vi "Set_Sweep_Parameter.vi"(5 "MPM":refnum<k24>[](array[refnum]), 6 "布尔":bool, 7 "OSU":refnum<k24>, 8 "错误输入（无错误）":errorcluster, 9 "TSL_OSUport":dbl, 10 "TSLSweepItem":T1, 11 "SPU":refnum<k24>) -> (0 "错误输出":errorcluster, 1 "MPM out":refnum<k24>[](array[refnum]), 2 "OSU out":refnum<k24>, 3 "SPU out":refnum<k24>)   [LabVIEW 2017]
uses:
  D:/test/FULLband-sts/Fullband_Sample/DLL/InstrumentDLL.dll
  DLL/InstrumentDLL.dll
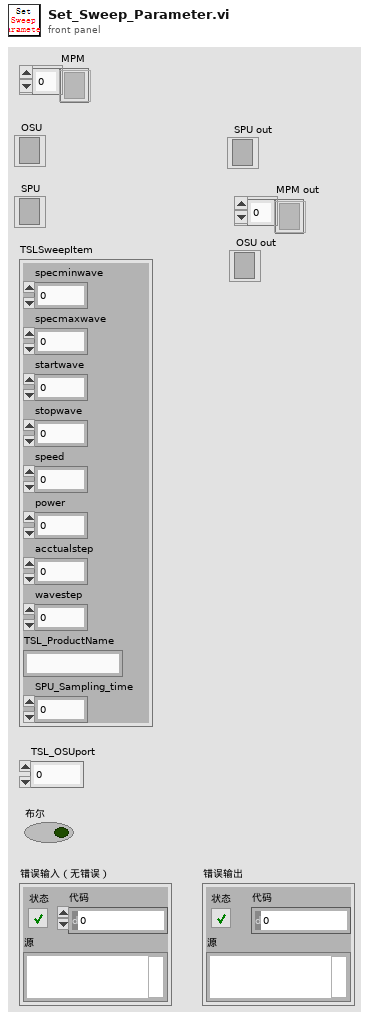
[diagram p1: front panel]
types:
  T1 = cluster{"specminwave":dbl, "specmaxwave":dbl, "startwave":dbl, "stopwave":dbl, "speed":dbl, "power":dbl, "acctualstep":dbl, "wavestep":dbl, "TSL_ProductName":string, "SPU_Sampling_time":dbl}
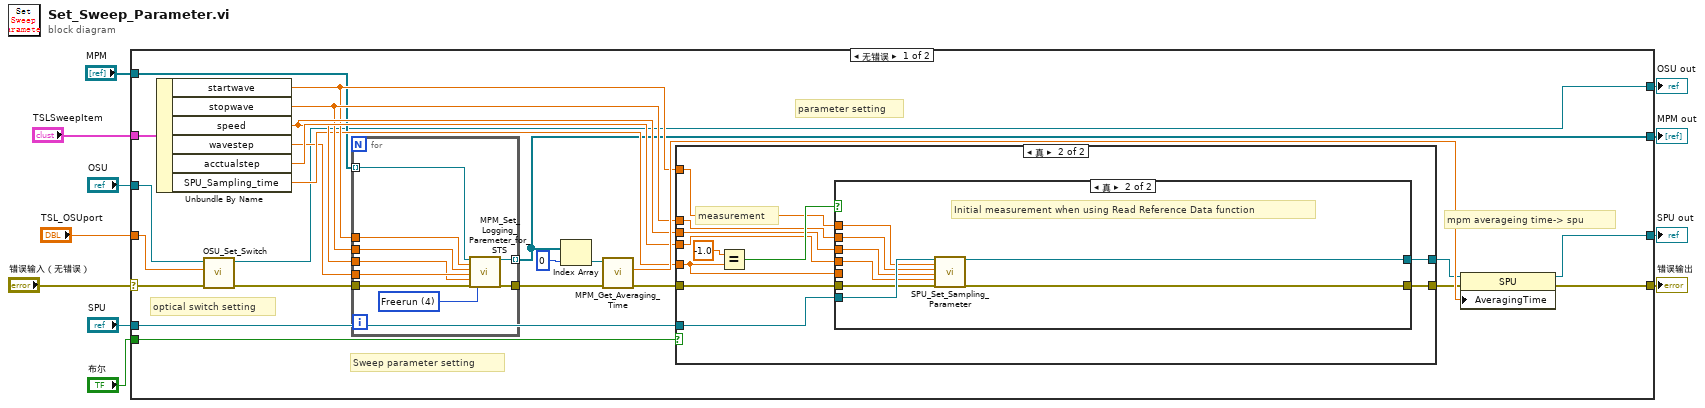
[diagram p0: block diagram]
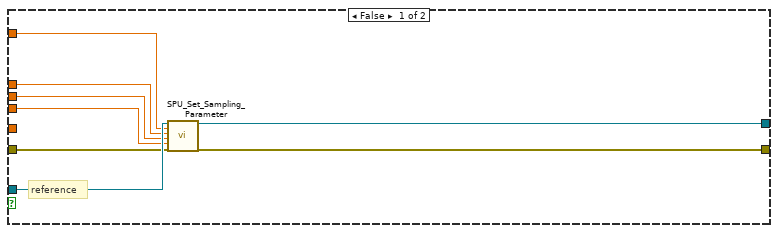
[diagram p2: hidden frame]
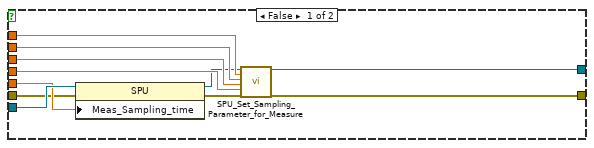
[diagram p3: hidden frame]
diagram:
  n1 = case shown="无错误" "错误输入（无错误）" {
    selector: "错误输入（无错误）" -> [w15 w87]
    tunnel: [w36 w87] -> w11
    tunnel: "SPU" -> [w27 w86]
    tunnel: "布尔" -> [w25 _]
    tunnel: "MPM" -> [w21 w84]
    tunnel: "TSL_OSUport" -> [w18 _]
    tunnel: "OSU" -> [w17 w85]
    tunnel: "TSLSweepItem" -> [w16 _]
    tunnel: [w14 w86] -> w3
    tunnel: [w13 w84] -> w2
    tunnel: [w12 w85] -> w1
    frame No Error {
      # "mpm averageing time-> spu"
      # "parameter setting"
      # "Sweep parameter setting"
      # "optical switch setting"
      n2 = Unbundle By Name(w16) -> ("startwave"=w29:dbl, "stopwave"=w30:dbl, "speed"=w31:dbl, "wavestep"=w20:dbl, "acctualstep"=w32:dbl, "SPU_Sampling_time"=w26:dbl)
      n3 = call "OSU_Set_Switch.vi"("error in (no error)"=w15, "channel"=w18, ".NET Reference in"=w17) -> ("error out"=w19:errorcluster, "Reference out"=w12:refnum<k24>)  [unwired: 7 in]
      n4 = for {
        tunnel: w19 -> [w83]
        tunnel: w21 -> [w82] mode=indexing
        tunnel: w29 -> [w81]
        tunnel: w30 -> [w80]
        tunnel: w20 -> [w79]
        tunnel: w31 -> [w78]
        tunnel: [w76] -> w24
        tunnel: [w75] -> w13 mode=indexing
        w77 = 4 items=["ManualRangeConstant", "ManualRangeSweep", "AutoRangeConstant", "AutoRangeSweep", "Freerun"] ("mode")
        n5 = call "MPM_Set_Logging_Paremeter_for_STS.vi"(".NET Reference in"=w82, "startwave"=w81, "stopwave"=w80, "wavestep"=w79, "speed"=w78, "error in (no error)"=w83, "mode"=w77) -> ("Reference out"=w75:refnum<k24>, "error out"=w76:errorcluster)  [unwired: 11 in]
      }
      n6 = Index Array(array=w13, index=0 ("索引")) -> (element=w23:refnum<k24>)
      n7 = call "MPM_Get_Averaging_Time.vi"("error in (no error)"=w24, ".NET Reference in"=w23) -> ("error out"=w28:errorcluster, "time out"=w35:dbl)  [unwired: 7 in, 1 out]
      n8 = case shown="真" w25 {
        tunnel: w26 -> [_ w46]
        tunnel: w27 -> [w44 w54]
        tunnel: w28 -> [w43 w50]
        tunnel: w29 -> [w42 w53]
        tunnel: w30 -> [w41 w49]
        tunnel: w31 -> [w40 w52]
        tunnel: w32 -> [w39 w51]
        tunnel: [w37 w48] -> w33
        tunnel: [w38 w47] -> w34
        frame False {
          # "reference"
          n9 = call "SPU_Set_Sampling_Parameter.vi"("引用"=w44, "startwave"=w42, "stopwave"=w41, "speed"=w40, "triggerstep"=w39, "错误输入（无错误）"=w43) -> ("引用输出"=w38:refnum<k24>, "error IO"=w37:errorcluster)  [unwired: 12 in]
        }
        frame True {
          # "measurement"
          n10 = Equal?(x=-1.0, y=w46) -> (x = y?=w55:bool)
          n11 = case shown="真" w55 {
            tunnel: w54 -> [w60 w74]
            tunnel: w53 -> [w66 w70]
            tunnel: w52 -> [w63 w71]
            tunnel: w51 -> [w65 w72]
            tunnel: w50 -> [w58 w73]
            tunnel: w49 -> [w64 w69]
            tunnel: [w61 w68] -> w48
            tunnel: [w62 w67] -> w47
            tunnel: w46 -> [w59 _]
            frame False {
              n12 = property on="属性节点" class="SPU"(reference=w60, error in=w58, "Meas_Sampling_time"=w59) -> (reference out=w57:refnum<k24>, error out=w56:errorcluster)
              n13 = call "SPU_Set_Sampling_Parameter_for_Measure.vi"("引用"=w57, "startwave"=w66, "stopwave"=w64, "speed"=w63, "triggerstep"=w65, "错误输入（无错误）"=w56) -> ("引用输出"=w62:refnum<k24>, "error IO"=w61:errorcluster)  [unwired: 12 in]
            }
            frame True {
              # "Initial measurement when using Read Reference Data function"
              n14 = call "SPU_Set_Sampling_Parameter.vi"("引用"=w74, "startwave"=w70, "stopwave"=w69, "speed"=w71, "triggerstep"=w72, "错误输入（无错误）"=w73) -> ("引用输出"=w67:refnum<k24>, "error IO"=w68:errorcluster)  [unwired: 12 in]
            }
          }
        }
      }
      n15 = property class="SPU"(reference=w34, error in=w33, "AveragingTime"=w35) -> (reference out=w14:refnum<k24>, error out=w36:errorcluster)
    }
    frame Error {
    }
  }
  "错误输出" <- w11
  "SPU out" <- w3
  "MPM out" <- w2
  "OSU out" <- w1
